vi "Translator.MainGui.vi"(6 "~Do not save font? (F)":bool, 8 "~error in":errorcluster, 9 "VI ref in [ ]":refnum<vi>[](array[refnum]), 10 "~Language in use":string="English", 11 "~Translation folder":path=path "D:/PL_0125_Sapphire_Automation_branches/SOFTWARE_v1.1-Translation/settings") -> (0 "~error out":errorcluster, 1 "~restart?":bool, 2 "~font name":string, 3 "VI ref out [ ]":refnum<vi>[](array[refnum]))   [LabVIEW 2019, in "Tools.lvlib"]
uses:
  Tools.lvlib
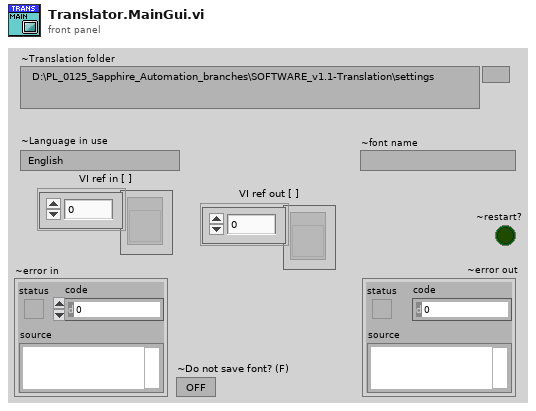
[diagram p1: front panel]
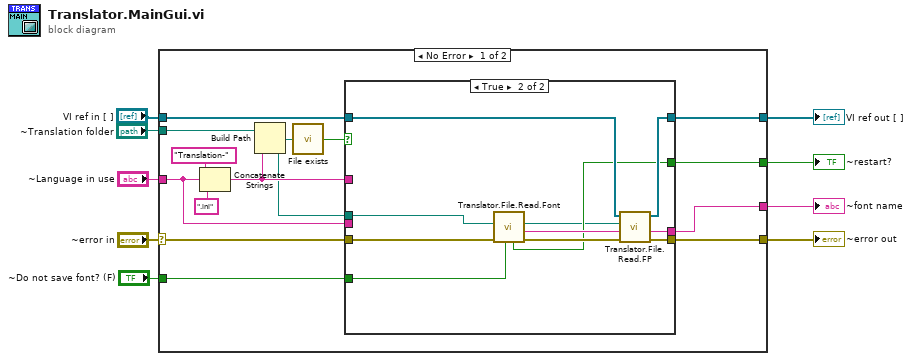
[diagram p0: block diagram]
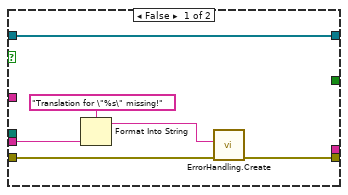
[diagram p2: hidden frame]
diagram:
  n1 = case shown="No Error" "~error in" {
    selector: "~error in" -> [w18 w41]
    tunnel: "~Translation folder" -> [w16 _]
    tunnel: [w14 w41] -> w6
    tunnel: "~Language in use" -> [w10 _]
    tunnel: [w15 _] -> w5
    tunnel: [w20 _] -> w4
    tunnel: "~Do not save font? (F)" -> [w17 _]
    tunnel: "VI ref in [ ]" -> [w12 w40]
    tunnel: [w11 w40] -> w1
    frame No Error {
      n2 = Concatenate Strings("Translation-" ("string"), w10, ".ini" ("string")) -> (w21:string)
      n3 = Build Path(base path=w16, name or relative path=w21) -> (appended path=w19:path)
      n4 = call "File exists.vi"("file path"=w19) -> ("exists?"=w13:bool)  [unwired: 4 in]
      n5 = case shown="True" w13 {
        tunnel: w18 -> [w28 w31]
        tunnel: [_ w39] -> w15
        tunnel: [w29 w30] -> w14
        tunnel: w19 -> [_ w34]
        tunnel: w21 -> [_ _]
        tunnel: [_ w33] -> w20
        tunnel: w17 -> [_ w38]
        tunnel: w12 -> [w25 w37]
        tunnel: [w25 w36] -> w11
        tunnel: w10 -> [w24 _]
        frame False {
          n6 = Format Into String(format string="Translation for \"%s\" missing!", w24) -> (resulting string=w26:string)  [unwired: 2 in, 1 out]
          n7 = call "ErrorHandling.Create.vi"("error in"=w28, "explanation"=w26) -> ("error out"=w29:errorcluster)  [unwired: 9 in]
        }
        frame True {
          n8 = call "Translator.File.Read.Font.vi"("Do not save font? (F)"=w38, "error in"=w31, "Translation file in"=w34) -> ("error out"=w35:errorcluster, "font name"=w39:string, "Translation file out"=w32:path, "restart required?"=w33:bool)  [unwired: 5 in]
          n9 = call "Translator.File.Read.FP.vi"("error in"=w35, "font name"=w39, "Translation file"=w32, "VI ref in [ ]"=w37) -> ("error out"=w30:errorcluster, "VI ref out [ ]"=w36:refnum<vi>[])  [unwired: 6 in]
        }
      }
    }
    frame Error {
    }
  }
  "~error out" <- w6
  "~font name" <- w5
  "~restart?" <- w4
  "VI ref out [ ]" <- w1
